vi "Main.vi"() -> ()   [LabVIEW 2016]
uses:
  <vilib>/Utility/error.llb/DialogType.ctl
  <vilib>/DAQmx/read.llb/DAQmx Read (Analog Wfm 1Chan 1Samp).vi
  <vilib>/DAQmx/miscellaneous.llb/DAQmx Fill In Error Info.vi
panel:
  in  "Input Terminal Configuration":T1(ring)
  in  "DAQ Physical Channel":tag
  out "Waveform Graph":waveform(dbl)(graph)
  in  "Samples Per Moving Average":i32=10
  in  "Voltage to AU Conversion Factor":dbl=1.0
  in  "Start":bool
  in  "Skip Export":bool
  in  "End Experiment?":bool
  in  "Export?":bool
  # "Set these values BEFORE starting \nthe experiment"
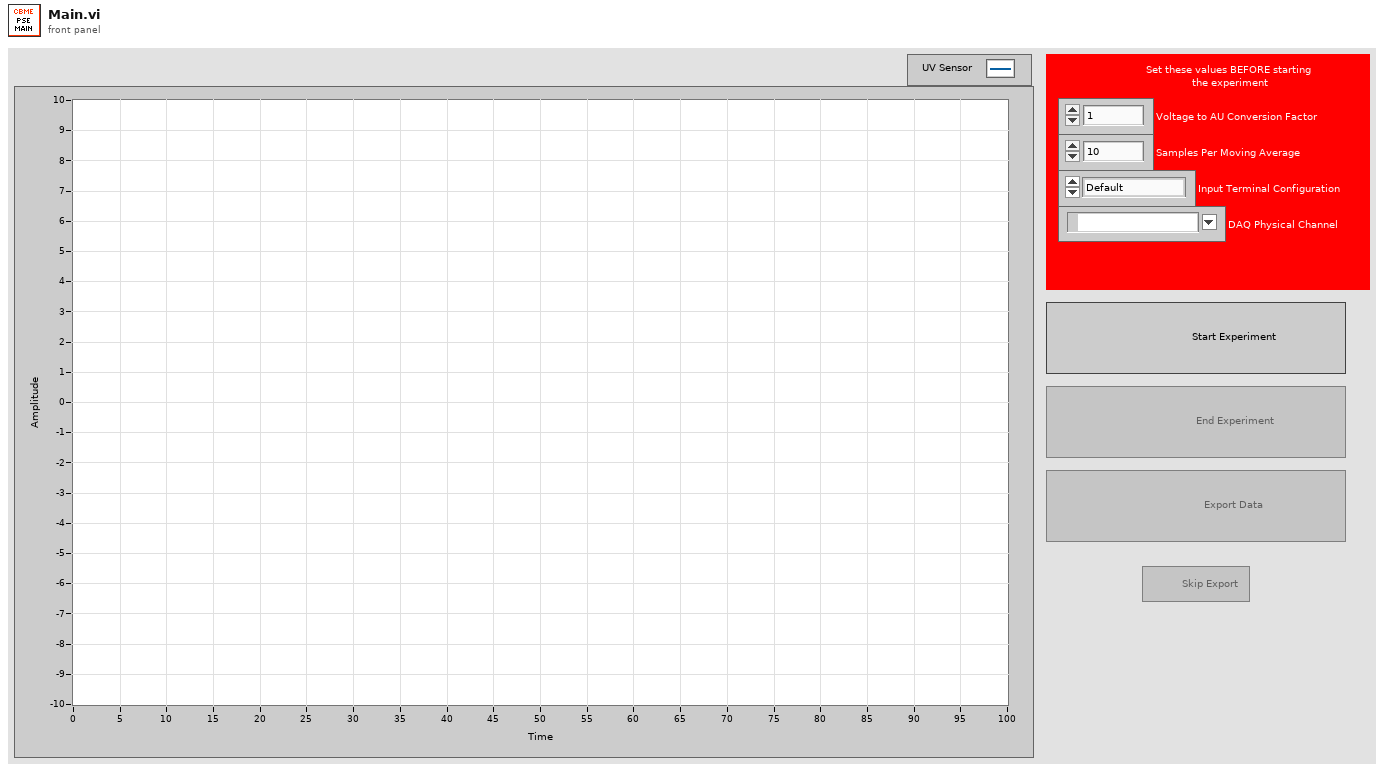
[diagram p1: front panel]
types:
  T1 = enum16{"Default", "RSE", "NRSE", "Differential", "Pseudodifferential"}
  T2 = enum8{"Enabled", "Disabled", "Disabled and Grayed Out"}
  T3 = typedef "DialogType.ctl" = u16
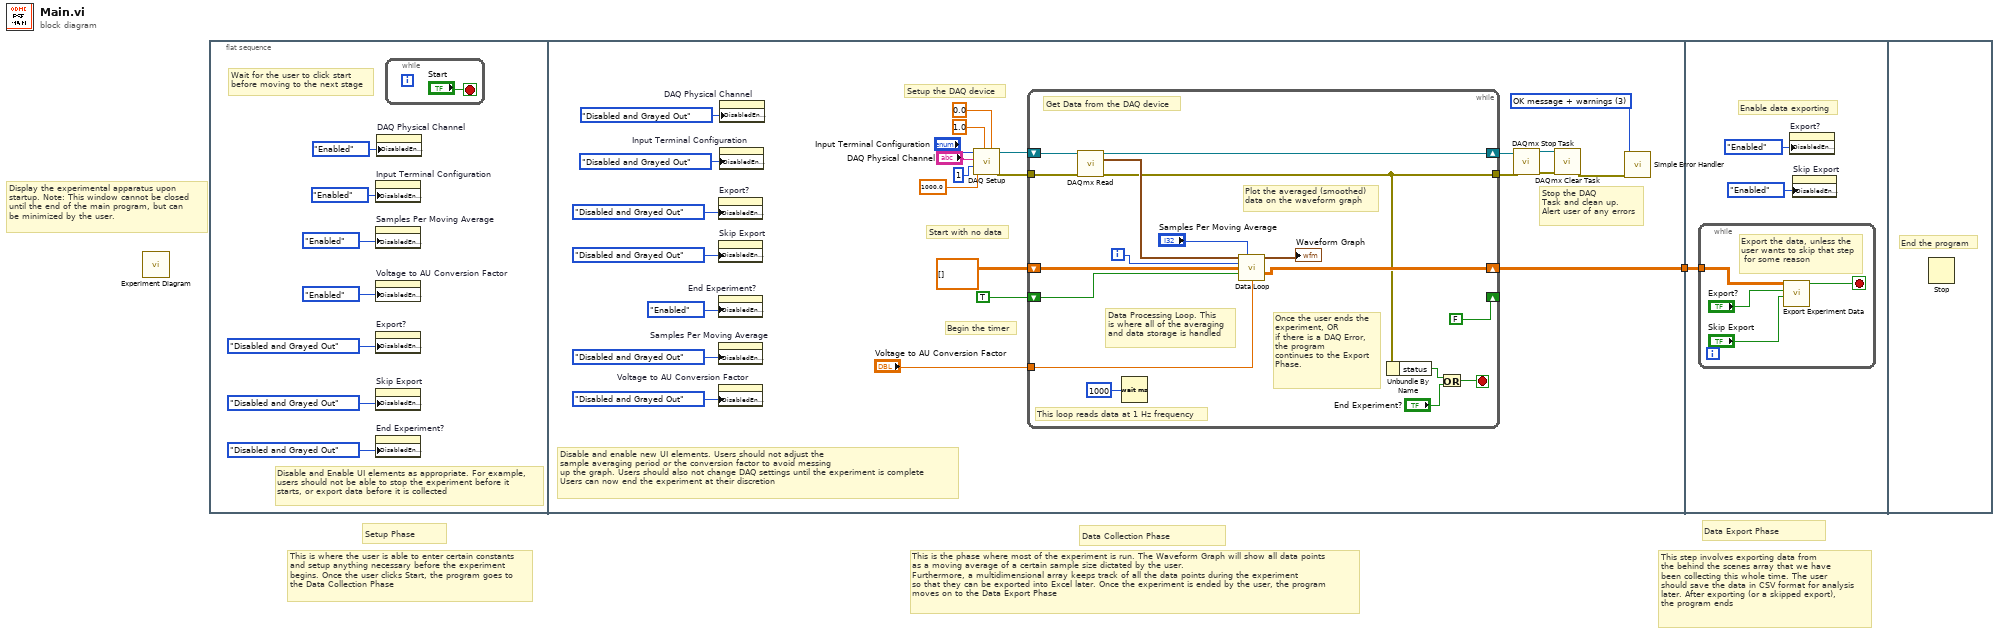
[diagram p0: block diagram]
diagram:
  # "This step involves exporting data from\nthe behind the scenes array that we have\nbeen collecting this whole time. The user \nshould save the data in CSV format for analysis \nlater. After exporting (or a skipped export),\nthe program ends"
  # "Data Export Phase"
  # "This is the phase where most of the experiment is run. The Waveform Graph will show all data points \nas a moving average of a certain sample size dictated by the user.\nFurthermore, a multidimensional array keeps track of all the data points during the experiment\nso that they can be exported into Excel later. Once the experiment is ended by the user, the program\nmoves on to the Data Export Phase"
  # "Data Collection Phase"
  # "This is where the user is able to enter certain constants\nand setup anything necessary before the experiment \nbegins. Once the user clicks Start, the program goes to\nthe Data Collection Phase"
  # "Setup Phase"
  # "Display the experimental apparatus upon\nstartup. Note: This window cannot be closed\nuntil the end of the main program, but can\nbe minimized by the user."
  n1 = call "Experiment Diagram.vi"() -> ()  [unwired: 12 in]
  n2 = flat-sequence {
    tunnel: [w30] -> w1
    tunnel: w1 -> [w52]
    frame #0 {
      # "Wait for the user to click start \nbefore moving to the next stage"
      # "Disable and Enable UI elements as appropriate. For example,\nusers should not be able to stop the experiment before it \nstarts, or export data before it is collected"
      n3 = property on="Input Terminal Configuration" class="Enum (strict)"("DisabledEnum"=T2."Enabled" ("Disabled")) -> ()  [unwired: 2 in, 2 out]
      n4 = property on="Samples Per Moving Average" class="DigNum (strict)"("DisabledEnum"=T2."Enabled" ("Disabled")) -> ()  [unwired: 2 in, 2 out]
      n5 = property on="Voltage to AU Conversion Factor" class="DigNum (strict)"("DisabledEnum"=T2."Enabled" ("Disabled")) -> ()  [unwired: 2 in, 2 out]
      n6 = property on="Export?" class="Bool"("DisabledEnum"=T2."Disabled and Grayed Out" ("Disabled")) -> ()  [unwired: 2 in, 2 out]
      n7 = property on="Skip Export" class="Bool"("DisabledEnum"=T2."Disabled and Grayed Out" ("Disabled")) -> ()  [unwired: 2 in, 2 out]
      n8 = property on="End Experiment?" class="Bool"("DisabledEnum"=T2."Disabled and Grayed Out" ("Disabled")) -> ()  [unwired: 2 in, 2 out]
      n9 = property on="DAQ Physical Channel" class="DAQmxName"("DisabledEnum"=T2."Enabled" ("Disabled")) -> ()  [unwired: 2 in, 2 out]
      n10 = while {
        stop <- "Start" stop-if-true
      }
    }
    frame #1 {
      w10 = T3 3 items=["no dialog", "OK message", "continue or stop message", "OK message + warnings", "continue/stop + warnings"] ("type of dialog (OK msg:1)")
      # "Stop the DAQ \nTask and clean up.\nAlert user of any errors"
      # "Start with no data"
      # "Begin the timer"
      # "Setup the DAQ device"
      # "Disable and enable new UI elements. Users should not adjust the\nsample averaging period or the conversion factor to avoid messing \nup the graph. Users should also not change DAQ settings until the experiment is complete\nUsers can now end the experiment at their discretion"
      n11 = property on="Export?" class="Bool"("DisabledEnum"=T2."Disabled and Grayed Out" ("Disabled")) -> ()  [unwired: 2 in, 2 out]
      n12 = property on="Skip Export" class="Bool"("DisabledEnum"=T2."Disabled and Grayed Out" ("Disabled")) -> ()  [unwired: 2 in, 2 out]
      n13 = property on="End Experiment?" class="Bool"("DisabledEnum"=T2."Enabled" ("Disabled")) -> ()  [unwired: 2 in, 2 out]
      n14 = property on="Samples Per Moving Average" class="DigNum (strict)"("DisabledEnum"=T2."Disabled and Grayed Out" ("Disabled")) -> ()  [unwired: 2 in, 2 out]
      n15 = property on="Voltage to AU Conversion Factor" class="DigNum (strict)"("DisabledEnum"=T2."Disabled and Grayed Out" ("Disabled")) -> ()  [unwired: 2 in, 2 out]
      n16 = property on="Input Terminal Configuration" class="Enum (strict)"("DisabledEnum"=T2."Disabled and Grayed Out" ("Disabled")) -> ()  [unwired: 2 in, 2 out]
      n17 = property on="DAQ Physical Channel" class="DAQmxName"("DisabledEnum"=T2."Disabled and Grayed Out" ("Disabled")) -> ()  [unwired: 2 in, 2 out]
      n18 = call "DAQ Setup.vi"("minimum value"=0.0, "maximum value"=1.0, "rate"=1000.0, "samples per channel"=1, "physical channel"="DAQ Physical Channel", "input terminal configuration"="Input Terminal Configuration") -> ("error out"=w24:errorcluster, "task out"=w25:refnum<k21>)  [unwired: 4 in]
      n19 = while {
        shift-right: [w50] -> w15
        shift-left: w25 -> [w51]
        shift-right: [FALSE] -> _
        shift-left: TRUE -> [w48]
        shift-right: [w46] -> w30
        shift-left: dbl[][] [] -> [w47]
        tunnel: "Voltage to AU Conversion Factor" -> [w45]
        tunnel: w24 -> [w40]
        tunnel: [w38] -> w12
        i -> [w44]
        stop <- w35 stop-if-true
        # "Data Processing Loop. This \nis where all of the averaging \nand data storage is handled"
        # "Plot the averaged (smoothed)\ndata on the waveform graph"
        # "Once the user ends the \nexperiment, OR\nif there is a DAQ Error,\nthe program \ncontinues to the Export\nPhase."
        # "This loop reads data at 1 Hz frequency"
        # "Get Data from the DAQ device"
        n20 = call-poly <vilib>:"DAQmx Read.vi"("task/channels in"=w51, "error in"=w40) -> ("task out"=w50:refnum<k21>, "data"=w41:waveform(dbl), "error out"=w38:errorcluster)  [unwired: 11 in]
        n21 = Wait (ms)(milliseconds to wait=u32 1000) -> ()  [unwired: 1 out]
        n22 = call "Data Loop.vi"("Waveform Data"=w41, "Samples Per Average"="Samples Per Moving Average", "Index"=w44, "Data Array in"=w47, "Reset?"=w48, "Voltage to AU Conversion Factor"=w45) -> ("Waveform Data 2"=→"Waveform Graph":waveform(dbl), "Data Array out"=w46:dbl[][])  [unwired: 8 in]
        n23 = Unbundle By Name(w38) -> ("status"=w37:bool)
        n24 = Or(x=w37, y="End Experiment?") -> (x .or. y?=w35:bool)
      }
      n25 = call <vilib>:"DAQmx Stop Task.vi"("task/channels in"=w15, "error in"=w12) -> ("task out"=w14:refnum<k21>, "error out"=w13:errorcluster)  [unwired: 12 in]
      n26 = call <vilib>:"DAQmx Clear Task.vi"("task in"=w14, "error in"=w13) -> ("error out"=w11:errorcluster)  [unwired: 13 in]
      n27 = call <vilib>:"Simple Error Handler.vi"("type of dialog (OK msg:1)"=w10, "error in (no error)"=w11) -> ()  [unwired: 3 in, 5 out]
    }
    frame #2 {
      # "Enable data exporting"
      n28 = while {
        tunnel: w52 -> [w58]
        stop <- w55 stop-if-true
        # "Export the data, unless the \nuser wants to skip that step\n for some reason"
        n29 = call "Export Experiment Data.vi"("Skip Export"="Skip Export", "Export?"="Export?", "Data"=w58) -> ("Export Complete?"=w55:bool)  [unwired: 8 in]
      }
      n30 = property on="Export?" class="Bool"("DisabledEnum"=T2."Enabled" ("Disabled")) -> ()  [unwired: 2 in, 2 out]
      n31 = property on="Skip Export" class="Bool"("DisabledEnum"=T2."Enabled" ("Disabled")) -> ()  [unwired: 2 in, 2 out]
    }
    frame #3 {
      # "End the program"
      n32 = Stop() -> ()  [unwired: 1 in]
    }
  }
